vi "sv_Bandpass Filter for a Range.vi"(8 "error in (no error)":errorcluster, 10 "harmonic range":cluster{"start":dbl, "stop":dbl}={"start"=-1.0, "stop"=-1.0} {"stop" format="%.2f"; "start" format="%.2f"}, 11 "fs":dbl=10.0) -> (0 "error out":errorcluster, 2 "delay [samples]":i32, 3 "FIR filter":dbl[](array[numeric]))   [LabVIEW 2017, in "SoundVib_ContSweptSine.lvlib"]
uses:
  <vilib>/addons/Sound and Vibration/svt_Continuous Swept Sine/SoundVib_ContSweptSine.lvlib
  <vilib>/addons/Sound and Vibration/svt_Continuous Swept Sine/subVIs/sv_Continuous Swept-Sine Errors.ctl
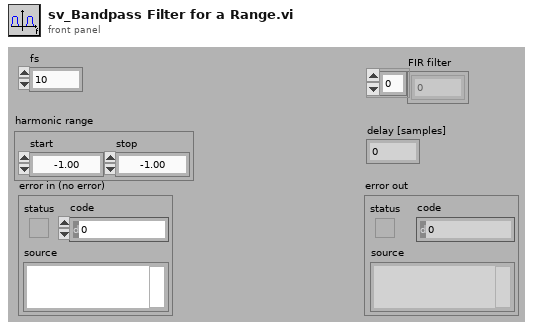
[diagram p1: front panel]
types:
  T1 = typedef "SoundVib_ContSweptSine.lvlib/sv_Continuous Swept-Sine Errors.ctl" = enum16{"Invalid AI sampling rate", "Item not found", "Invalid initial phase"}
  T2 = enum32{"Lowpass", "Highpass", "Bandpass", "Bandstop"}
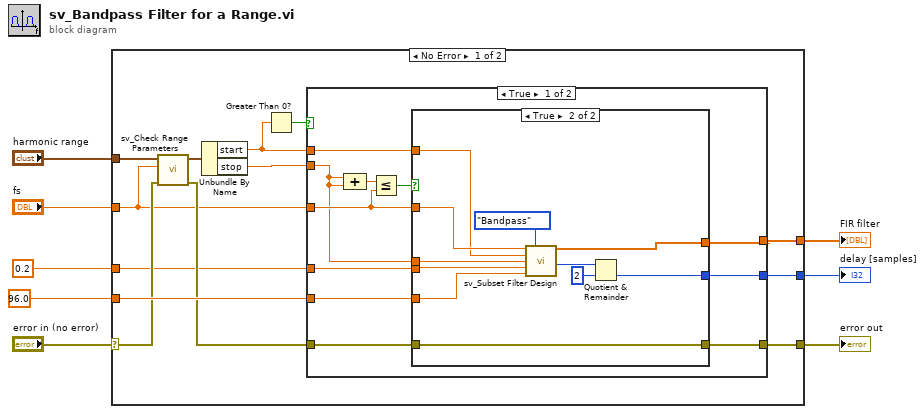
[diagram p0: block diagram]
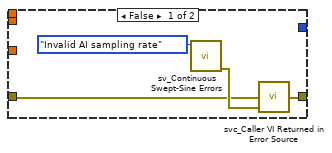
[diagram p2: hidden frame]
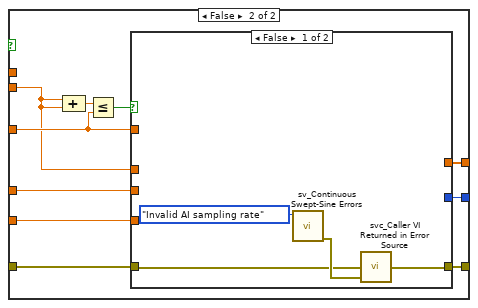
[diagram p3: hidden frame]
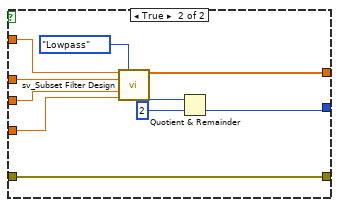
[diagram p4: hidden frame]
diagram:
  n1 = case shown="No Error" "error in (no error)" {
    selector: "error in (no error)" -> [w16 w72]
    tunnel: 0.2 ("passband") -> [w11 _]
    tunnel: 96.0 ("A stop [dB]") -> [w21 _]
    tunnel: [w20 _] -> w6
    tunnel: [w19 _] -> w5
    tunnel: "fs" -> [w12 _]
    tunnel: "harmonic range" -> [w14 _]
    tunnel: [w18 w72] -> w2
    frame No Error {
      n2 = call <vilib>:"sv_Check Range Parameters.vi"("error in (no error)"=w16, "fs"=w12, "harmonic range"=w14) -> ("error out"=w15:errorcluster, "harmonic range out"=w13:cluster{"start":dbl, "stop":dbl})  [unwired: 6 in, 1 out]
      n3 = Unbundle By Name(w13) -> ("start"=w9:dbl, "stop"=w17:dbl)
      n4 = Greater Than 0?(x=w9) -> (x > 0?=w10:bool)
      n5 = case shown="True" w10 {
        tunnel: w21 -> [w32 w57]
        tunnel: [w31 w56] -> w20
        tunnel: [w30 w55] -> w19
        tunnel: [w28 w53] -> w18
        tunnel: w17 -> [w23 w48]
        tunnel: w15 -> [w26 w51]
        tunnel: w12 -> [w25 w50]
        tunnel: w9 -> [w22 _]
        tunnel: w11 -> [w24 w49]
        frame True {
          n6 = Compound Arithmetic op=ADD(w23, w23) -> (w27:dbl)
          n7 = Less Or Equal?(x=w27, y=w25) -> (x <= y?=w29:bool)
          n8 = case shown="True" w29 {
            tunnel: w32 -> [_ w47]
            tunnel: [_ w44] -> w31
            tunnel: [_ w41] -> w30
            tunnel: w25 -> [_ w43]
            tunnel: w26 -> [w33 w42]
            tunnel: [w35 w42] -> w28
            tunnel: w24 -> [_ w40]
            tunnel: w23 -> [_ w39]
            tunnel: w22 -> [_ w38]
            frame False {
              n9 = call <vilib>:"sv_Continuous Swept-Sine Errors.vi"("continuous swept-sine error"=sv_Continuous_Swept-Sine_Errors."Invalid AI sampling rate") -> ("error out"=w34:errorcluster)  [unwired: 10 in]
              n10 = call <vilib>:"svc_Caller VI Returned in Error Source.vi"("warning input to caller"=w34, "error in (no error)"=w33) -> ("error out"=w35:errorcluster)  [unwired: 3 in]
            }
            frame True {
              n11 = call <vilib>:"sv_Subset Filter Design.vi"("fs"=w43, "filter type"=T2."Bandpass", "fl"=w38, "fh"=w39, "delta f"=w40, "A stop [dB]"=w47) -> ("filter coefficients"=w41:dbl[], "taps"=w45:i32)  [unwired: 7 in, 1 out]
              n12 = Quotient & Remainder(x=w45, y=2) -> (floor(x/y)=w44:i32)  [unwired: 1 out]
            }
          }
        }
        frame False {
          n13 = Compound Arithmetic op=ADD(w48, w48) -> (w52:dbl)
          n14 = Less Or Equal?(x=w52, y=w50) -> (x <= y?=w54:bool)
          n15 = case shown="False" w54 {
            tunnel: w57 -> [_ w71]
            tunnel: [_ w68] -> w56
            tunnel: [_ w65] -> w55
            tunnel: w50 -> [_ w67]
            tunnel: w51 -> [w58 w66]
            tunnel: [w60 w66] -> w53
            tunnel: w49 -> [_ w64]
            tunnel: w48 -> [_ w63]
            frame False {
              n16 = call <vilib>:"sv_Continuous Swept-Sine Errors.vi"("continuous swept-sine error"=sv_Continuous_Swept-Sine_Errors."Invalid AI sampling rate") -> ("error out"=w59:errorcluster)  [unwired: 10 in]
              n17 = call <vilib>:"svc_Caller VI Returned in Error Source.vi"("warning input to caller"=w59, "error in (no error)"=w58) -> ("error out"=w60:errorcluster)  [unwired: 3 in]
            }
            frame True {
              n18 = call <vilib>:"sv_Subset Filter Design.vi"("fs"=w67, "filter type"=T2."Lowpass", "fl"=w63, "delta f"=w64, "A stop [dB]"=w71) -> ("filter coefficients"=w65:dbl[], "taps"=w69:i32)  [unwired: 8 in, 1 out]
              n19 = Quotient & Remainder(x=w69, y=2) -> (floor(x/y)=w68:i32)  [unwired: 1 out]
            }
          }
        }
      }
    }
    frame Error {
    }
  }
  "delay [samples]" <- w6
  "FIR filter" <- w5
  "error out" <- w2
